vi "4_Math_loop.vi"() -> ()   [LabVIEW 2023]
panel:
  out "OUT MathScript":dbl=76.0
  in  "stop":bool
  out "OUT Formula":dbl=76.0
  in  "a":dbl=1.0
  in  "x":dbl=5.0
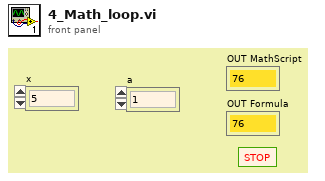
[diagram p1: front panel]
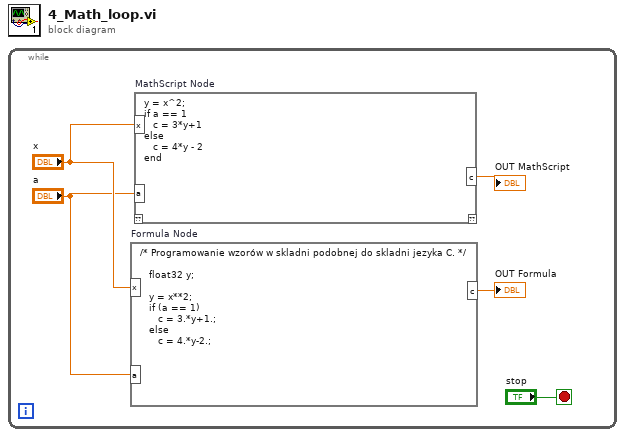
[diagram p0: block diagram]
diagram:
  n1 = while {
    stop <- "stop" stop-if-true
    n2 = formula code="/* Programowanie wzorów w skladni podobnej do skladni jezyka C. */\n\n   float32 y;\n\n   y = x**2;\n   if (a == 1) \n      c = 3.*y+1.;\n   else\n      c = 4.*y-2.;"("x"="x", "a"="a") -> ("c"=→"OUT Formula":dbl)
    n3 = mathscript code="y = x^2;\nif a == 1\n   c = 3*y+1\nelse\n   c = 4*y - 2\nend"("x"="x", "a"="a") -> ("c"=→"OUT MathScript":dbl)  [unwired: 1 in, 1 out]
  }
